vi "ResAcc data filter test.vi"() -> ()   [LabVIEW 2013]
panel:
  out "웨이브폼 그래프 2":dynamicdata(graph)=[{"t0"=timestamp(3537480678.7124343 s since 1904-01-01), "dt"=1.0, "Y"=array[2000 elements], "attributes"=variant("NI_ChannelName"=variant(string "필터된"))}, {"t0"=timestamp(3537480678.7124343 s since 1904-01-01), "dt"=1.0, "Y"=array[2000 elements], "attributes"=variant("NI_ChannelName"=variant(string "필터된"))}, {"t0"=timestamp(3537480678.7124343 s since 1904-01-01), "dt"=1.0, "Y"=array[2000 elements], "attributes"=variant("NI_ChannelName"=variant(string "필터된"))}, {"t0"=timestamp(3537480678.7124343 s since 1904-01-01), "dt"=1.0, "Y"=array[2000 elements], "attributes"=variant("NI_ChannelName"=variant(string "필터된"))}, {"t0"=timestamp(3537480678.7124343 s since 1904-01-01), "dt"=1.0, "Y"=array[2000 elements], "attributes"=variant("NI_ChannelName"=variant(string "필터된"))}, {"t0"=timestamp(3537480678.7124343 s since 1904-01-01), "dt"=1.0, "Y"=array[2000 elements], "attributes"=variant("NI_ChannelName"=variant(string "필터된"))}, {"t0"=timestamp(3537480678.7124343 s since 1904-01-01), "dt"=1.0, "Y"=array[2000 elements], "attributes"=variant("NI_ChannelName"=variant(string "필터된"))}, {"t0"=timestamp(3537480678.7124343 s since 1904-01-01), "dt"=1.0, "Y"=array[2000 elements], "attributes"=variant("NI_ChannelName"=variant(string "필터된"))}, {"t0"=timestamp(3537480678.7124343 s since 1904-01-01), "dt"=1.0, "Y"=array[2000 elements], "attributes"=variant("NI_ChannelName"=variant(string "필터된"))}, {"t0"=timestamp(3537480678.7124343 s since 1904-01-01), "dt"=1.0, "Y"=array[2000 elements], "attributes"=variant("NI_ChannelName"=variant(string "필터된"))}, {"t0"=timestamp(3537480678.7124343 s since 1904-01-01), "dt"=1.0, "Y"=array[2000 elements], "attributes"=variant("NI_ChannelName"=variant(string "필터된"))}, {"t0"=timestamp(3537480678.7124343 s since 1904-01-01), "dt"=1.0, "Y"=array[2000 elements], "attributes"=variant("NI_ChannelName"=variant(string "필터된"))}, {"t0"=timestamp(3537480678.7124343 s since 1904-01-01), "dt"=1.0, "Y"=array[2000 elements], "attributes"=variant("NI_ChannelName"=variant(string "필터된"))}, {"t0"=timestamp(3537480678.7124343 s since 1904-01-01), "dt"=1.0, "Y"=array[2000 elements], "attributes"=variant("NI_ChannelName"=variant(string "필터된"))}, {"t0"=timestamp(3537480678.7124343 s since 1904-01-01), "dt"=1.0, "Y"=array[2000 elements], "attributes"=variant("NI_ChannelName"=variant(string "필터된"))}, {"t0"=timestamp(3537480678.7124343 s since 1904-01-01), "dt"=1.0, "Y"=array[2000 elements], "attributes"=variant("NI_ChannelName"=variant(string "필터된"))}]
  out "웨이브폼 그래프":dynamicdata(graph)=[{"t0"=timestamp(3537480678.7124343 s since 1904-01-01), "dt"=1.0, "Y"=array[2000 elements]}, {"t0"=timestamp(3537480678.7124343 s since 1904-01-01), "dt"=1.0, "Y"=array[2000 elements]}, {"t0"=timestamp(3537480678.7124343 s since 1904-01-01), "dt"=1.0, "Y"=array[2000 elements]}, {"t0"=timestamp(3537480678.7124343 s since 1904-01-01), "dt"=1.0, "Y"=array[2000 elements]}, {"t0"=timestamp(3537480678.7124343 s since 1904-01-01), "dt"=1.0, "Y"=array[2000 elements]}, {"t0"=timestamp(3537480678.7124343 s since 1904-01-01), "dt"=1.0, "Y"=array[2000 elements]}, {"t0"=timestamp(3537480678.7124343 s since 1904-01-01), "dt"=1.0, "Y"=array[2000 elements]}, {"t0"=timestamp(3537480678.7124343 s since 1904-01-01), "dt"=1.0, "Y"=array[2000 elements]}, {"t0"=timestamp(3537480678.7124343 s since 1904-01-01), "dt"=1.0, "Y"=array[2000 elements]}, {"t0"=timestamp(3537480678.7124343 s since 1904-01-01), "dt"=1.0, "Y"=array[2000 elements]}, {"t0"=timestamp(3537480678.7124343 s since 1904-01-01), "dt"=1.0, "Y"=array[2000 elements]}, {"t0"=timestamp(3537480678.7124343 s since 1904-01-01), "dt"=1.0, "Y"=array[2000 elements]}, {"t0"=timestamp(3537480678.7124343 s since 1904-01-01), "dt"=1.0, "Y"=array[2000 elements]}, {"t0"=timestamp(3537480678.7124343 s since 1904-01-01), "dt"=1.0, "Y"=array[2000 elements]}, {"t0"=timestamp(3537480678.7124343 s since 1904-01-01), "dt"=1.0, "Y"=array[2000 elements]}, {"t0"=timestamp(3537480678.7124343 s since 1904-01-01), "dt"=1.0, "Y"=array[2000 elements]}]
  in  "Acc&Res":dbl[][](array[numeric])=array16x2000[32000 elements] caption="가속도, 저항" format="%#.2p"
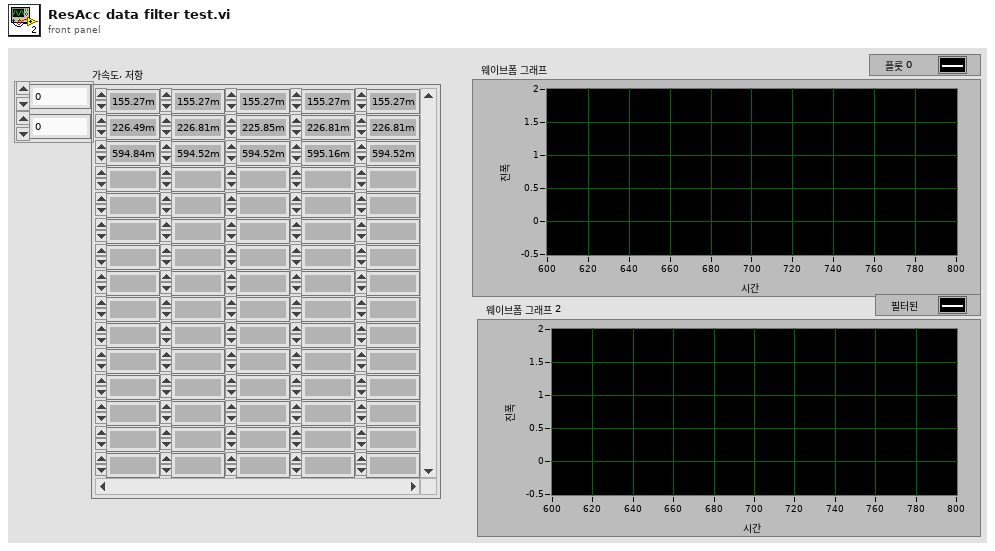
[diagram p1: front panel]
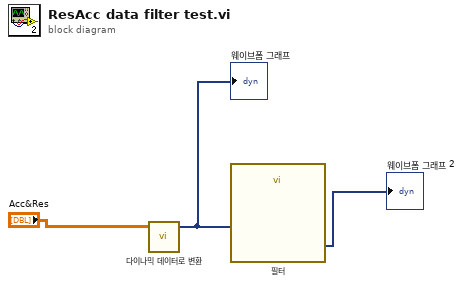
[diagram p0: block diagram]
diagram:
  n1 = call "다이나믹 데이터로 변환"("2D Array"="Acc&Res") -> ("Dynamic Data Type"=w2:dynamicdata)  [unwired: 3 in]
  "웨이브폼 그래프" <- w2
  n2 = call "필터"("Signal"=w2) -> ("Filtered Signal"=→"웨이브폼 그래프 2":dynamicdata)  [unwired: 9 in, 1 out]
